vi "HEWH Calcs.vi"(6 "Calculate?":bool, 9 "Save Terms":T1) -> (1 "Read Terms":T1)   [LabVIEW 2009]
uses:
  Terms_HEWH Computations.ctl
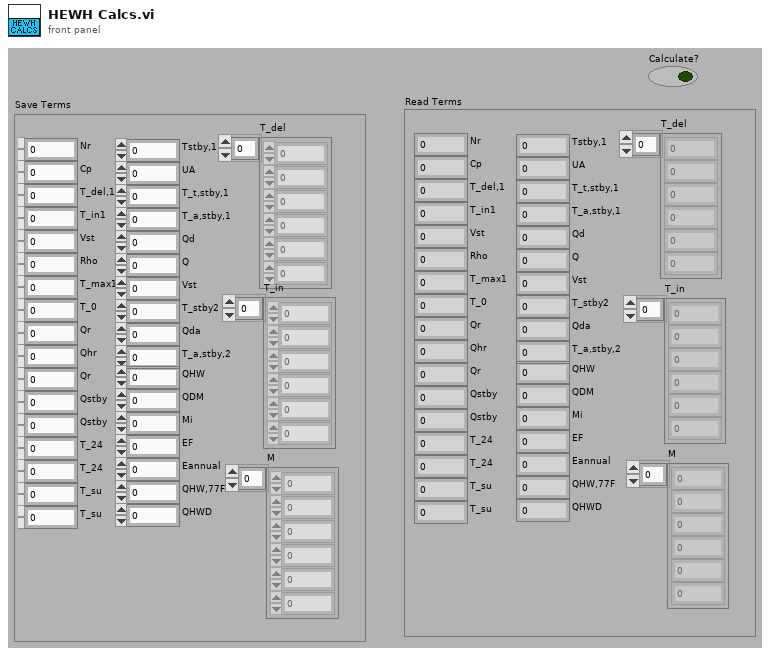
[diagram p1: front panel]
types:
  T1 = typedef "Terms_HEWH Computations.ctl" = cluster{"Cp":dbl, "T_del,1":dbl, "T_in1":dbl, "Qr":dbl, "Vst":dbl, "Rho":dbl, "T_max1":dbl, "T_0":dbl, "Nr":dbl, "Qstby":dbl, "T_24":dbl, "T_su":dbl, "Qhr":dbl, "Qstby":dbl, "T_24":dbl, "T_su":dbl, "Qr":dbl, "Tstby,1":dbl, "UA":dbl, "T_t,stby,1":dbl, "T_a,stby,1":dbl, "Qd":dbl, "Q":dbl, "Vst":dbl, "T_stby2":dbl, "Qda":dbl, "T_a,stby,2":dbl, "QHW":dbl, "Mi":dbl, "T_del":dbl[], "T_in":dbl[], "M":dbl[], "QHW,77F":dbl, "QHWD":dbl, "QDM":dbl, "EF":dbl, "Eannual":dbl}
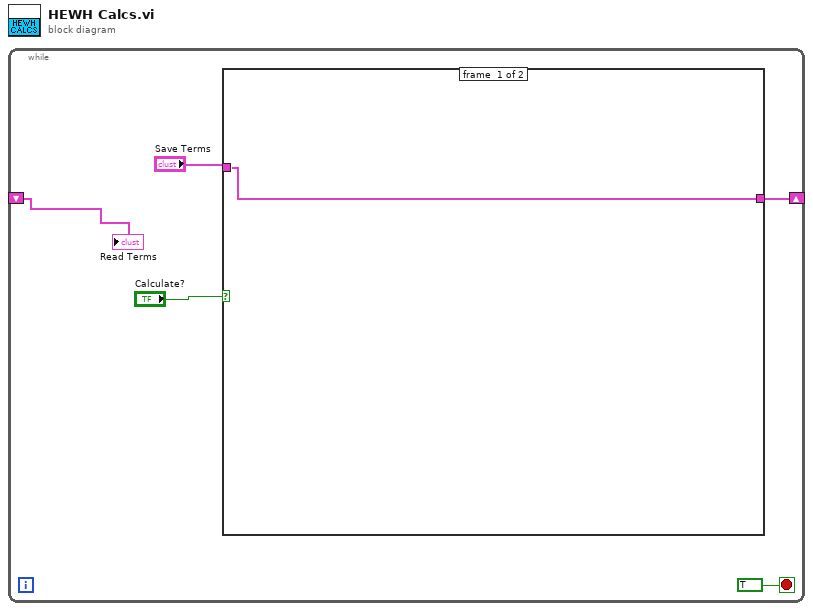
[diagram p0: block diagram]
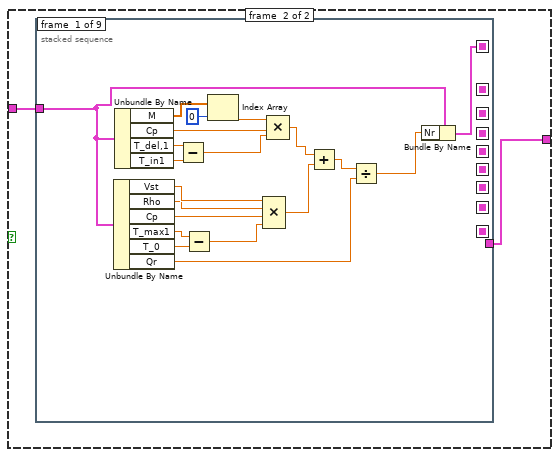
[diagram p2: hidden frame]
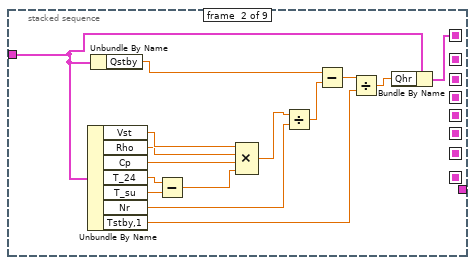
[diagram p3: hidden frame]
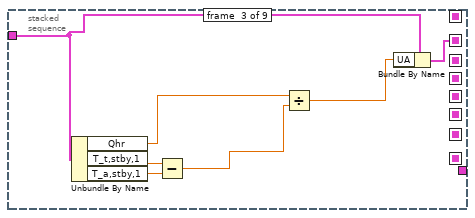
[diagram p4: hidden frame]
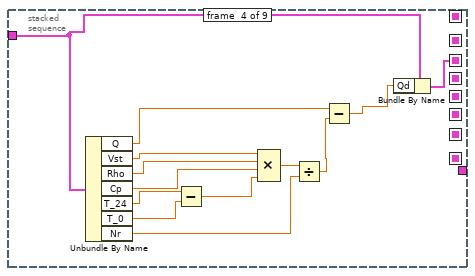
[diagram p5: hidden frame]
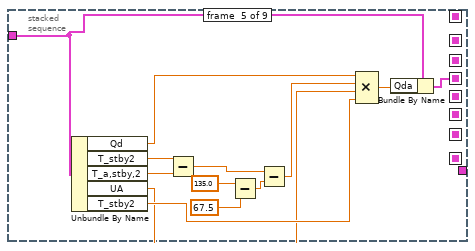
[diagram p6: hidden frame]
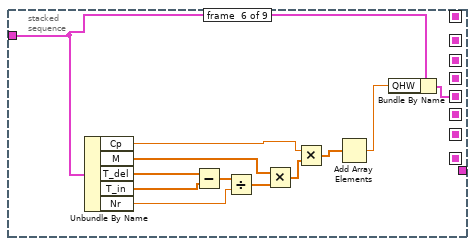
[diagram p7: hidden frame]
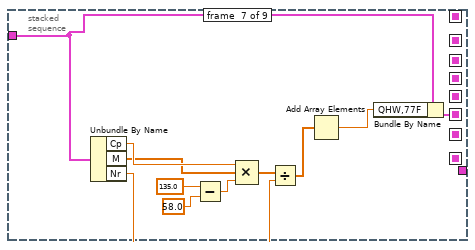
[diagram p8: hidden frame]
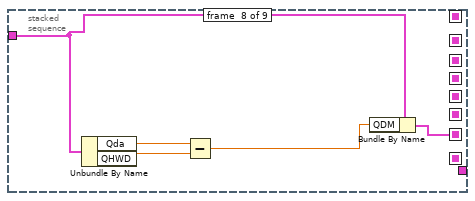
[diagram p9: hidden frame]
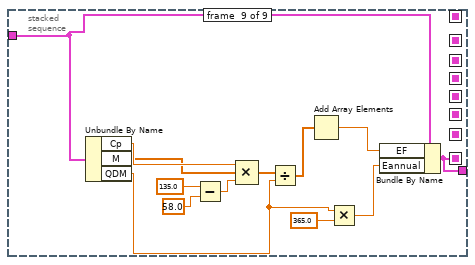
[diagram p10: hidden frame]
diagram:
  n1 = while {
    shift-right: [w4] -> _
    shift-left: _ -> [w1]
    stop <- TRUE stop-if-true
    n2 = case shown="True" "Calculate?" {
      tunnel: "Save Terms" -> [w6 w8]
      tunnel: [w6 w7] -> w4
      frame #0 {
      }
      frame #1 {
        n3 = stacked-sequence {
          seq-local: [w9 _ _ _ _ _ _ _ _] -> [_ _ _ _ _ _ _ _ _]
          seq-local: [_ w29 _ _ _ _ _ _ _] -> [_ _ _ _ _ _ _ _ _]
          seq-local: [_ _ w44 _ _ _ _ _ _] -> [_ _ _ _ _ _ _ _ _]
          seq-local: [_ _ _ w51 _ _ _ _ _] -> [_ _ _ _ _ _ _ _ _]
          seq-local: [_ _ _ _ w64 _ _ _ _] -> [_ _ _ _ _ _ _ _ _]
          seq-local: [_ _ _ _ _ w77 _ _ _] -> [_ _ _ _ _ _ _ _ _]
          seq-local: [_ _ _ _ _ _ w98 _ _] -> [_ _ _ _ _ _ _ _ _]
          seq-local: [_ _ _ _ _ _ _ w103 _] -> [_ _ _ _ _ _ _ _ _]
          seq-local: [_ _ _ _ _ _ _ _ w105] -> [_ _ _ _ _ _ _ _ _]
          tunnel: w8 -> [w28 w43 w50 w63 w76 w88 w99 w104 w117]
          tunnel: [_ _ _ _ _ _ _ _ w105] -> w7
          frame #0 {
            n4 = Unbundle By Name(w28) -> ("Vst"=w18:dbl, "Rho"=w17:dbl, "Cp"=w16:dbl, "T_max1"=w20:dbl, "T_0"=w19:dbl, "Qr"=w11:dbl)
            n5 = Unbundle By Name(w28) -> ("M"=w27:dbl[], "Cp"=w22:dbl, "T_del,1"=w25:dbl, "T_in1"=w24:dbl)
            n6 = Subtract(x=w25, y=w24) -> (x-y=w21:dbl)
            n7 = Subtract(x=w20, y=w19) -> (x-y=w15:dbl)
            n8 = Index Array(array=w27, index=0) -> (element=w23:dbl)
            n9 = Compound Arithmetic op=MULTIPLY(w18, w17, w16, w15) -> (w13:dbl)
            n10 = Compound Arithmetic op=MULTIPLY(w23, w22, w21) -> (w14:dbl)
            n11 = Add(x=w14, y=w13) -> (x+y=w12:dbl)
            n12 = Divide(x=w12, y=w11) -> (x/y=w10:dbl)
            n13 = Bundle By Name(cluster=w28, "Nr"=w10) -> (w9:T1)
          }
          frame #1 {
            n14 = Unbundle By Name(w43) -> ("Vst"=w40:dbl, "Rho"=w39:dbl, "Cp"=w38:dbl, "T_24"=w42:dbl, "T_su"=w41:dbl, "Nr"=w36:dbl, "Tstby,1"=w31:dbl)
            n15 = Unbundle By Name(w43) -> ("Qstby"=w34:dbl)
            n16 = Subtract(x=w42, y=w41) -> (x-y=w37:dbl)
            n17 = Compound Arithmetic op=MULTIPLY(w40, w39, w38, w37) -> (w35:dbl)
            n18 = Divide(x=w35, y=w36) -> (x/y=w33:dbl)
            n19 = Subtract(x=w34, y=w33) -> (x-y=w32:dbl)
            n20 = Divide(x=w32, y=w31) -> (x/y=w30:dbl)
            n21 = Bundle By Name(cluster=w43, "Qhr"=w30) -> (w29:T1)
          }
          frame #2 {
            n22 = Unbundle By Name(w50) -> ("Qhr"=w47:dbl, "T_t,stby,1"=w49:dbl, "T_a,stby,1"=w48:dbl)
            n23 = Subtract(x=w49, y=w48) -> (x-y=w46:dbl)
            n24 = Divide(x=w47, y=w46) -> (x/y=w45:dbl)
            n25 = Bundle By Name(cluster=w50, "UA"=w45) -> (w44:T1)
          }
          frame #3 {
            n26 = Unbundle By Name(w63) -> ("Q"=w61:dbl, "Vst"=w59:dbl, "Rho"=w58:dbl, "Cp"=w57:dbl, "T_24"=w56:dbl, "T_0"=w55:dbl, "Nr"=w53:dbl)
            n27 = Subtract(x=w56, y=w55) -> (x-y=w54:dbl)
            n28 = Compound Arithmetic op=MULTIPLY(w59, w58, w57, w54) -> (w62:dbl)
            n29 = Divide(x=w62, y=w53) -> (x/y=w60:dbl)
            n30 = Subtract(x=w61, y=w60) -> (x-y=w52:dbl)
            n31 = Bundle By Name(cluster=w63, "Qd"=w52) -> (w51:T1)
          }
          frame #4 {
            n32 = Unbundle By Name(w76) -> ("Qd"=w65:dbl, "T_stby2"=w71:dbl, "T_a,stby,2"=w70:dbl, "UA"=w67:dbl, "T_stby2"=w68:dbl)
            n33 = Subtract(x=w71, y=w70) -> (x-y=w69:dbl)
            n34 = Subtract(x=135.0, y=67.5) -> (x-y=w72:dbl)
            n35 = Subtract(x=w69, y=w72) -> (x-y=w66:dbl)
            n36 = Compound Arithmetic op=MULTIPLY(w65, w66, w67, w68) -> (w75:dbl)
            n37 = Bundle By Name(cluster=w76, "Qda"=w75) -> (w64:T1)
          }
          frame #5 {
            n38 = Unbundle By Name(w88) -> ("Cp"=w83:dbl, "M"=w80:dbl[], "T_del"=w87:dbl[], "T_in"=w86:dbl[], "Nr"=w84:dbl)
            n39 = Subtract(x=w87, y=w86) -> (x-y=w85:dbl[])
            n40 = Divide(x=w85, y=w84) -> (x/y=w81:dbl[])
            n41 = Multiply(x=w80, y=w81) -> (x*y=w82:dbl[])
            n42 = Multiply(x=w83, y=w82) -> (x*y=w79:dbl[])
            n43 = Add Array Elements(numeric array=w79) -> (sum=w78:dbl)
            n44 = Bundle By Name(cluster=w88, "QHW"=w78) -> (w77:T1)
          }
          frame #6 {
            n45 = Unbundle By Name(w99) -> ("Cp"=w93:dbl, "M"=w92:dbl[], "Nr"=w90:dbl)
            n46 = Subtract(x=135.0, y=58.0) -> (x-y=w94:dbl)
            n47 = Compound Arithmetic op=MULTIPLY(w93, w92, w94) -> (w91:dbl[])
            n48 = Divide(x=w91, y=w90) -> (x/y=w89:dbl[])
            n49 = Add Array Elements(numeric array=w89) -> (sum=w97:dbl)
            n50 = Bundle By Name(cluster=w99, "QHW,77F"=w97) -> (w98:T1)
          }
          frame #7 {
            n51 = Unbundle By Name(w104) -> ("Qda"=w102:dbl, "QHWD"=w101:dbl)
            n52 = Subtract(x=w102, y=w101) -> (x-y=w100:dbl)
            n53 = Bundle By Name(cluster=w104, "QDM"=w100) -> (w103:T1)
          }
          frame #8 {
            n54 = Unbundle By Name(w117) -> ("Cp"=w112:dbl, "M"=w111:dbl[], "QDM"=w107:dbl)
            n55 = Subtract(x=135.0, y=58.0) -> (x-y=w113:dbl)
            n56 = Compound Arithmetic op=MULTIPLY(w112, w111, w113) -> (w110:dbl[])
            n57 = Divide(x=w110, y=w107) -> (x/y=w109:dbl[])
            n58 = Add Array Elements(numeric array=w109) -> (sum=w116:dbl)
            n59 = Multiply(x=w107, y=365.0) -> (x*y=w106:dbl)
            n60 = Bundle By Name(cluster=w117, "EF"=w116, "Eannual"=w106) -> (w105:T1)
          }
        }
      }
    }
    "Read Terms" <- w1
  }
